vi "nameTaps.vi"() -> ()   [LabVIEW 2011]
panel:
  out "Array":string[](array[string])=["Path", "Boolean", "String", "ComboBox", "String", "Boolean", "Boolean", "String", "Enum", "TabControl", "String", "Cluster", "Digital", "Digital"]
  in  "vi path":path=path "C:/Users/loasis/Documents/000 LabView/Developers Version/Interface/GUI_TRA_NEW/GUI_TRA_NEW.vi"
  in  "position::1":dbl=3.42565 min=0.0 max=6.0
  in  "X":T1={"Channel::1"=enum."Axis 3"}
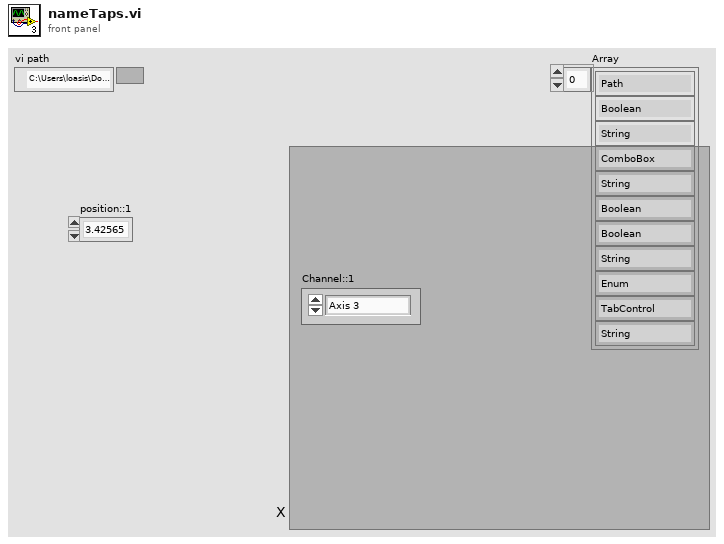
[diagram p1: front panel]
types:
  T1 = cluster{"Channel::1":enum16{"Axis 1", "Axis 3", "Axis 5"}}
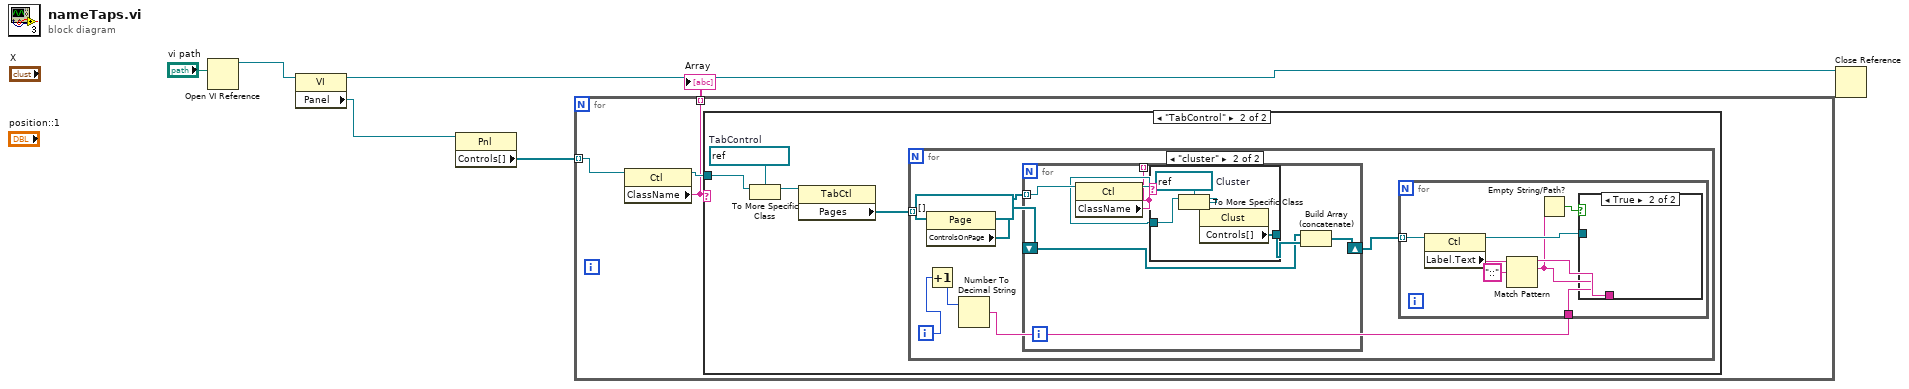
[diagram p0: block diagram]
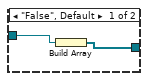
[diagram p3: hidden frame]
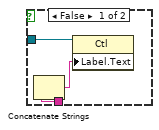
[diagram p4: hidden frame]
diagram:
  n1 = Open VI Reference(vi path="vi path") -> (vi reference=w5:refnum<vi>)  [unwired: 5 in, 1 out]
  n2 = property class="VI"(reference=w5) -> (reference out=w2:refnum<vi>, "Panel"=w4:refnum<vi>)  [unwired: 1 in, 1 out]
  n3 = property class="Pnl"(reference=w4) -> ("Controls[]"=w3:refnum<vi>[])  [unwired: 1 in, 2 out]
  n4 = for {
    tunnel: w3 -> [w9] mode=indexing
    tunnel: [w7] -> w1 mode=indexing
    n5 = property class="Ctl"(reference=w9) -> (reference out=w8:refnum<vi>, "ClassName"=w7:string)  [unwired: 1 in, 1 out]
    n6 = case shown="\"TabControl\"" w7 {
      tunnel: w8 -> [_ w13]
      frame "False", Default {
      }
      frame "TabControl" {
        w12 = refnum<vi> refnum  # TabControl
        n7 = To More Specific Class(target class=w12, reference=w13) -> (specific class reference=w11:refnum<vi>)  [unwired: 1 in, 1 out]
        n8 = property class="TabCtl"(reference=w11) -> ("Pages"=w10:refnum<vi>[])  [unwired: 1 in, 2 out]
        n9 = for {
          tunnel: w10 -> [w20] mode=indexing
          i -> [w15]
          n10 = property class="Page"(reference=w20) -> ("ControlsOnPage"=w18:refnum<vi>[])  [unwired: 1 in, 2 out]
          n11 = Increment(x=w15) -> (x+1=w14:i32)
          n12 = Number To Decimal String(number=w14) -> (decimal integer string=w19:string)  [unwired: 1 in]
          n13 = for {
            tunnel: w18 -> [w26] mode=indexing
            shift-right: [w23] -> w16
            shift-left: refnum<vi>[] [] -> [w22]
            tunnel: [w21] -> _ mode=indexing
            n14 = property class="Ctl"(reference=w26) -> (reference out=w25:refnum<vi>, "ClassName"=w21:string)  [unwired: 1 in, 1 out]
            n15 = case shown="\"cluster\"" w21 {
              tunnel: w25 -> [w28 w32]
              tunnel: [w27 w29] -> w24
              frame "False", Default {
                n16 = Build Array(w28) -> (w27:refnum<vi>[])
              }
              frame "cluster" {
                w30 = refnum<vi> refnum  # Cluster
                n17 = To More Specific Class(target class=w30, reference=w32) -> (specific class reference=w31:refnum<vi>)  [unwired: 1 in, 1 out]
                n18 = property class="Clust"(reference=w31) -> ("Controls[]"=w29:refnum<vi>[])  [unwired: 1 in, 2 out]
              }
            }
            n19 = Build Array (concatenate)(w22, w24) -> (w23:refnum<vi>[])
          }
          n20 = for {
            tunnel: w16 -> [w40] mode=indexing
            tunnel: w19 -> [w36]
            n21 = property class="Ctl"(reference=w40) -> (reference out=w35:refnum<vi>, "Label.Text"=w39:string)  [unwired: 1 in, 1 out]
            n22 = Match Pattern(string=w39, regular expression="::") -> (before substring=w37:string, match substring=w34:string)  [unwired: 1 in, 2 out]
            n23 = Empty String/Path?(string/path=w34) -> (empty?=w33:bool)
            n24 = case shown="True" w33 {
              tunnel: w37 -> [w45 _]
              tunnel: w36 -> [w44 _]
              tunnel: w35 -> [w43 _]
              tunnel: w34 -> [w41 _]
              frame False {
                n25 = Concatenate Strings(w45, w41, w44) -> (w42:string)
                n26 = property class="Ctl"(reference=w43, "Label.Text"=w42) -> ()  [unwired: 1 in, 2 out]
              }
              frame True {
              }
            }
          }
        }
      }
    }
  }
  "Array" <- w1
  n27 = Close Reference(reference=w2) -> ()  [unwired: 1 in, 1 out]
